vi "Weather Parse Test.vi"() -> ()   [LabVIEW 2020, in "CDM-Config.lvlib"] (continued)
the average of the highest one-\\nthird of the combined wind-wave and swell height.\\n\\n.TONIGHT...NE winds 40 kt. Blowing snow.\\n.WED...NE winds 35 kt.\\n.WED NIGHT...NE winds 30 kt.\\n.THU...NE winds 20 kt.\\n.THU NIGHT...NE winds 20 kt.\\n.FRI...NE winds 20 kt.\\n.FRI NIGHT...NE winds 20 kt.\\n.SAT...NE winds 30 kt.\\n.SUN...NE winds 40 kt.\",\n                \"instruction\": null,\n                \"response\": \"Avoid\",\n                \"parameters\": {\n                    \"AWIPSidentifier\": [\n                        \"CWFWCZ\"\n                    ],\n                    \"WMOidentifier\": [\n                        \"FZAK52 PAFG 030049\"\n                    ],\n                    \"NWSheadline\": [\n                        \"GALE WARNING IN EFFECT THROUGH WEDNESDAY MORNING\"\n                    ],\n                    \"BLOCKCHANNEL\": [\n                        \"EAS\",\n                        \"NWEM\",\n                        \"CMAS\"\n                    ],\n                    \"VTEC\": [\n                        \"/O.NEW.PAFG.GL.W.2010.251203T0000Z-251204T0200Z/\"\n                    ],\n                    \"eventEndingTime\": [\n                        \"2025-12-03T17:00:00-09:00\"\n                    ]\n                },\n                \"scope\": \"Public\",\n                \"code\": \"IPAWSv1.0\",\n                \"language\": \"en-US\",\n                \"web\": \"http://www.weather.gov\",\n                \"eventCode\": {\n                    \"SAME\": [\n                        \"NWS\"\n                    ],\n                    \"NationalWeatherService\": [\n                        \"GLW\"\n                    ]\n                }\n            }\n        },\n        {\n            \"id\": \"https://api.weather.gov/alerts/urn:oid:2.49.0.1.840.0.52fef07b0c3a98d88109cd1837a99c72cb982c5b.007.1\",\n            \"type\": \"Feature\",\n            \"geometry\": null,\n            \"properties\": {\n                \"@id\": \"https://api.weather.gov/alerts/urn:oid:2.49.0.1.840.0.52fef07b0c3a98d88109cd1837a99c72cb982c5b.007.1\",\n                \"@type\": \"wx:Alert\",\n                \"id\": \"urn:oid:2.49.0.1.840.0.52fef07b0c3a98d88109cd1837a99c72cb982c5b.007.1\",\n                \"areaDesc\": \"Wales to Cape Espenberg out to 15 NM\",\n                \"geocode\": {\n                    \"SAME\": [\n                        \"058807\"\n                    ],\n                    \"UGC\": [\n                        \"PKZ807\"\n                    ]\n                },\n                \"affectedZones\": [\n                    \"https://api.weather.gov/zones/forecast/PKZ807\"\n                ],\n                \"references\": [],\n                \"sent\": \"2025-12-02T15:49:00-09:00\",\n                \"effective\": \"2025-12-02T15:49:00-09:00\",\n                \"onset\": \"2025-12-02T15:00:00-09:00\",\n                \"expires\": \"2025-12-03T06:00:00-09:00\",\n                \"ends\": \"2025-12-03T17:00:00-09:00\",\n                \"status\": \"Actual\",\n                \"messageType\": \"Alert\",\n                \"category\": \"Met\",\n                \"severity\": \"Minor\",\n                \"certainty\": \"Likely\",\n                \"urgency\": \"Expected\",\n                \"event\": \"Brisk Wind Advisory\",\n                \"sender\": \"w-nws.webmaster@noaa.gov\",\n                \"senderName\": \"NWS Fairbanks AK\",\n                \"headline\": \"Brisk Wind Advisory issued December 2 at 3:49PM AKST until December 3 at 5:00PM AKST by NWS Fairbanks AK\",\n                \"description\": \"Northwestern Alaska Coastal Waters out 100 NM\\n\\nWind forecasts reflect the predominant speed and direction\\nexpected. Sea forecasts represent the average of the highest one-\\nthird of the combined wind-wave and swell height.\\n\\n.TONIGHT...N winds 30 kt.\\n.WED...N winds 25 kt.\\n.WED NIGHT...SE winds 10 kt.\\n.THU...SE winds 10 kt.\\n.THU NIGHT...E winds 10 kt.\\n.FRI...NE winds 10 kt.\\n.FRI NIGHT...NE winds 15 kt.\\n.SAT...NE winds 25 kt.\\n.SUN...NE winds 30 kt.\",\n                \"instruction\": null,\n                \"response\": \"Avoid\",\n                \"parameters\": {\n                    \"AWIPSidentifier\": [\n                        \"CWFWCZ\"\n                    ],\n                    \"WMOidentifier\": [\n                        \"FZAK52 PAFG 030049\"\n                    ],\n                    \"NWSheadline\": [\n                        \"BRISK WIND ADVISORY IN EFFECT THROUGH WEDNESDAY MORNING\"\n                    ],\n                    \"BLOCKCHANNEL\": [\n                        \"EAS\",\n                        \"NWEM\",\n                        \"CMAS\"\n                    ],\n                    \"VTEC\": [\n                        \"/O.NEW.PAFG.BW.Y.2013.251203T0000Z-251204T0200Z/\"\n                    ],\n                    \"eventEndingTime\": [\n                        \"2025-12-03T17:00:00-09:00\"\n                    ]\n                },\n                \"scope\": \"Public\",\n                \"code\": \"IPAWSv1.0\",\n                \"language\": \"en-US\",\n                \"web\": \"http://www.weather.gov\",\n                \"eventCode\": {\n                    \"SAME\": [\n                        \"NWS\"\n                    ],\n                    \"NationalWeatherService\": [\n                        \"BWY\"\n                    ]\n                }\n            }\n        },\n        {\n            \"id\": \"https://api.weather.gov/alerts/urn:oid:2.49.0.1.840.0.52fef07b0c3a98d88109cd1837a99c72cb982c5b.014.2\",\n            \"type\": \"Feature\",\n            \"geometry\": null,\n            \"properties\": {\n                \"@id\": \"https://api.weather.gov/alerts/urn:oid:2.49.0.1.840.0.52fef07b0c3a98d88109cd1837a99c72cb982c5b.014.2\",\n                \"@type\": \"wx:Alert\",\n                \"id\": \"urn:oid:2.49.0.1.840.0.52fef07b0c3a98d88109cd1837a99c72cb982c5b.014.2\",\n                \"areaDesc\": \"Southwest of Saint Lawrence Island from 15 to 100 NM\",\n                \"geocode\": {\n                    \"SAME\": [\n                        \"058851\"\n                    ],\n                    \"UGC\": [\n                        \"PKZ851\"\n                    ]\n                },\n                \"affectedZones\": [\n                    \"https://api.weather.gov/zones/forecast/PKZ851\"\n                ],\n                \"references\": [],\n                \"sent\": \"2025-12-02T15:49:00-09:00\",\n                \"effective\": \"2025-12-02T15:49:00-09:00\",\n                \"onset\": \"2025-12-02T15:00:00-09:00\",\n                \"expires\": \"2025-12-03T06:00:00-09:00\",\n                \"ends\": \"2025-12-03T17:00:00-09:00\",\n                \"status\": \"Actual\",\n                \"messageType\": \"Alert\",\n                \"category\": \"Met\",\n                \"severity\": \"Severe\",\n                \"certainty\": \"Likely\",\n                \"urgency\": \"Expected\",\n                \"event\": \"Heavy Freezing Spray Warning\",\n                \"sender\": \"w-nws.webmaster@noaa.gov\",\n                \"senderName\": \"NWS Fairbanks AK\",\n                \"headline\": \"Heavy Freezing Spray Warning issued December 2 at 3:49PM AKST until December 3 at 5:00PM AKST by NWS Fairbanks AK\",\n                \"description\": \"Northwestern Alaska Coastal Waters out 100 NM\\n\\nWind forecasts reflect the predominant speed and direction\\nexpected. Sea forecasts represent the average of the highest one-\\nthird of the combined wind-wave and swell height.\\n\\n.TONIGHT...NE winds 40 kt. Seas 13 ft. Heavy freezing spray.\\n.WED...NE winds 35 kt. Seas 10 ft. Heavy freezing spray.\\n.WED NIGHT...N winds 25 kt. Seas 6 ft. Heavy freezing spray.\\n.THU...NE winds 20 kt. Seas 4 ft. Freezing spray.\\n.THU NIGHT...NE winds 20 kt. Seas 4 ft. Heavy freezing spray.\\n.FRI...NE winds 20 kt. Seas 9 ft. Heavy freezing spray.\\n.FRI NIGHT...NE winds 20 kt. Seas 9 ft. Freezing spray.\\n.SAT...NE winds 25 kt. Seas 12 ft.\\n.SUN...NE winds 35 kt. Seas 14 ft.\",\n                \"instruction\": null,\n                \"response\": \"Avoid\",\n                \"parameters\": {\n                    \"AWIPSidentifier\": [\n                        \"CWFWCZ\"\n                    ],\n                    \"WMOidentifier\": [\n                        \"FZAK52 PAFG 030049\"\n                    ],\n                    \"NWSheadline\": [\n                        \"GALE WARNING IN EFFECT THROUGH WEDNESDAY MORNING... ...HEAVY FREEZING SPRAY WARNING IN EFFECT THROUGH WEDNESDAY AFTERNOON\"\n                    ],\n                    \"BLOCKCHANNEL\": [\n                        \"EAS\",\n                        \"NWEM\",\n                        \"CMAS\"\n                    ],\n                    \"VTEC\": [\n                        \"/O.NEW.PAFG.UP.W.2021.251203T0000Z-251204T0200Z/\"\n                    ],\n                    \"eventEndingTime\": [\n                        \"2025-12-03T17:00:00-09:00\"\n                    ]\n                },\n                \"scope\": \"Public\",\n                \"code\": \"IPAWSv1.0\",\n                \"language\": \"en-US\",\n                \"web\": \"http://www.weather.gov\",\n                \"eventCode\": {\n                    \"SAME\": [\n                        \"NWS\"\n                    ],\n                    \"NationalWeatherService\": [\n                        \"UPW\"\n                    ]\n                }\n            }\n        },\n        {\n            \"id\": \"https://api.weather.gov/alerts/urn:oid:2.49.0.1.840.0.52fef07b0c3a98d88109cd1837a99c72cb982c5b.011.1\",\n            \"type\": \"Feature\",\n            \"geometry\": null,\n            \"properties\": {\n                \"@id\": \"https://api.weather.gov/alerts/urn:oid:2.49.0.1.840.0.52fef07b0c3a98d88109cd1837a99c72cb982c5b.011.1\",\n                \"@type\": \"wx:Alert\",\n                \"id\": \"urn:oid:2.49.0.1.840.0.52fef07b0c3a98d88109cd1837a99c72cb982c5b.011.1\",\n                \"areaDesc\": \"South Side of Saint Lawrence Island out to 15 NM\",\n                \"geocode\": {\n                    \"SAME\": [\n                        \"058816\"\n                    ],\n                    \"UGC\": [\n                        \"PKZ816\"\n                    ]\n                },\n                \"affectedZones\": [\n                    \"https://api.weather.gov/zones/forecast/PKZ816\"\n                ],\n                \"references\": [],\n                \"sent\": \"2025-12-02T15:49:00-09:00\",\n                \"effective\": \"2025-12-02T15:49:00-09:00\",\n                \"onset\": \"2025-12-02T15:00:00-09:00\",\n                \"expires\": \"2025-12-03T06:00:00-09:00\",\n                \"ends\": \"2025-12-03T17:00:00-09:00\",\n                \"status\": \"Actual\",\n                \"messageType\": \"Alert\",\n                \"category\": \"Met\",\n                \"severity\": \"Moderate\",\n                \"certainty\": \"Likely\",\n                \"urgency\": \"Expected\",\n                \"event\": \"Gale Warning\",\n                \"sender\": \"w-nws.webmaster@noaa.gov\",\n                \"senderName\": \"NWS Fairbanks AK\",\n                \"headline\": \"Gale Warning issued December 2 at 3:49PM AKST until December 3 at 5:00PM AKST by NWS Fairbanks AK\",\n                \"description\": \"Northwestern Alaska Coastal Waters out 100 NM\\n\\nWind forecasts reflect the predominant speed and direction\\nexpected. Sea forecasts represent the average of the highest one-\\nthird of the combined wind-wave and swell height.\\n\\n.TONIGHT...N winds 40 kt. Seas 10 ft. Heavy freezing spray.\\n.WED...N winds 35 kt. Seas 8 ft. Heavy freezing spray.\\n.WED NIGHT...N winds 25 kt. Seas 5 ft. Heavy freezing spray.\\n.THU...NE winds 15 kt. Seas 3 ft. Freezing spray.\\n.THU NIGHT...NE winds 15 kt. Seas 3 ft. Freezing spray.\\n.FRI...NE winds 15 kt. Seas 6 ft. Heavy freezing spray.\\n.FRI NIGHT...NE winds 20 kt. Seas 8 ft. Freezing spray.\\n.SAT...NE winds 25 kt. Seas 10 ft.\\n.SUN...NE winds 35 kt. Seas 10 ft.\",\n                \"instruction\": null,\n                \"response\": \"Avoid\",\n                \"parameters\": {\n                    \"AWIPSidentifier\": [\n                        \"CWFWCZ\"\n                    ],\n                    \"WMOidentifier\": [\n                        \"FZAK52 PAFG 030049\"\n                    ],\n                    \"NWSheadline\": [\n                        \"GALE WARNING IN EFFECT THROUGH WEDNESDAY MORNING... ...HEAVY FREEZING SPRAY WARNING IN EFFECT THROUGH WEDNESDAY AFTERNOON\"\n                    ],\n                    \"BLOCKCHANNEL\": [\n                        \"EAS\",\n                        \"NWEM\",\n                        \"CMAS\"\n                    ],\n                    \"VTEC\": [\n                        \"/O.NEW.PAFG.GL.W.2014.251203T0000Z-251204T0200Z/\"\n                    ],\n                    \"eventEndingTime\": [\n                        \"2025-12-03T17:00:00-09:00\"\n                    ]\n                },\n                \"scope\": \"Public\",\n                \"code\": \"IPAWSv1.0\",\n                \"language\": \"en-US\",\n                \"web\": \"http://www.weather.gov\",\n                \"eventCode\": {\n                    \"SAME\": [\n                        \"NWS\"\n                    ],\n                    \"NationalWeatherService\": [\n                        \"GLW\"\n                    ]\n                }\n            }\n        },\n        {\n            \"id\": \"https://api.weather.gov/alerts/urn:oid:2.49.0.1.840.0.52fef07b0c3a98d88109cd1837a99c72cb982c5b.006.2\",\n            \"type\": \"Feature\",\n            \"geometry\": null,\n            \"properties\": {\n                \"@id\": \"https://api.weather.gov/alerts/urn:oid:2.49.0.1.840.0.52fef07b0c3a98d88109cd1837a99c72cb982c5b.006.2\",\n                \"@type\": \"wx:Alert\",\n                \"id\": \"urn:oid:2.49.0.1.840.0.52fef07b0c3a98d88109cd1837a99c72cb982c5b.006.2\",\n                \"areaDesc\": \"Sledge Island to Wales out to 15 NM\",\n                \"geocode\": {\n                    \"SAME\": [\n                        \"058806\"\n                    ],\n                    \"UGC\": [\n                        \"PKZ806\"\n                    ]\n                },\n                \"affectedZones\": [\n                    \"https://api.weather.gov/zones/forecast/PKZ806\"\n                ],\n                \"references\": [],\n                \"sent\": \"2025-12-02T15:49:00-09:00\",\n                \"effective\": \"2025-12-02T15:49:00-09:00\",\n                \"onset\": \"2025-12-02T15:00:00-09:00\",\n                \"expires\": \"2025-12-03T06:00:00-09:00\",\n                \"ends\": \"2025-12-03T17:00:00-09:00\",\n                \"status\": \"Actual\",\n                \"messageType\": \"Alert\",\n                \"category\": \"Met\",\n                \"severity\": \"Severe\",\n                \"certainty\": \"Likely\",\n                \"urgency\": \"Expected\",\n                \"event\": \"Heavy Freezing Spray Warning\",\n                \"sender\": \"w-nws.webmaster@noaa.gov\",\n                \"senderName\": \"NWS Fairbanks AK\",\n                \"headline\": \"Heavy Freezing Spray Warning issued December 2 at 3:49PM AKST until December 3 at 5:00PM AKST by NWS Fairbanks AK\",\n                \"description\": \"Northwestern Alaska Coastal Waters out 100 NM\\n\\nWind forecasts reflect the predominant speed and direction\\nexpected. Sea forecasts represent the average of the highest one-\\nthird of the combined wind-wave and swell height.\\n\\n.TONIGHT...N winds 35 kt. Seas 7 ft. Heavy freezing spray.\\n.WED...N winds 35 kt. Seas 6 ft. Heavy freezing spray.\\n.WED NIGHT...NE winds 20 kt. Seas 3 ft. Heavy freezing spray.\\n.THU...NE winds 10 kt. Seas 1 foot.\\n.THU NIGHT...NE winds 10 kt. Seas 2 ft.\\n.FRI...NE winds 15 kt. Seas 3 ft. Heavy freezing spray.\\n.FRI NIGHT...NE winds 20 kt. Seas 5 ft. Heavy freezing spray.\\n.SAT...NE winds 25 kt. Seas 5 ft.\\n.SUN...NE winds 30 kt. Seas 6 ft.\",\n                \"instruction\": null,\n                \"response\": \"Avoid\",\n                \"parameters\": {\n                    \"AWIPSidentifier\": [\n                        \"CWFWCZ\"\n                    ],\n                    \"WMOidentifier\": [\n                        \"FZAK52 PAFG 030049\"\n                    ],\n                    \"NWSheadline\": [\n                        \"GALE WARNING IN EFFECT THROUGH LATE TONIGHT... ...HEAVY FREEZING SPRAY WARNING IN EFFECT THROUGH WEDNESDAY AFTERNOON\"\n                    ],\n                    \"BLOCKCHANNEL\": [\n                        \"EAS\",\n                        \"NWEM\",\n                        \"CMAS\"\n                    ],\n                    \"VTEC\": [\n                        \"/O.NEW.PAFG.UP.W.2012.251203T0000Z-251204T0200Z/\"\n                    ],\n                    \"eventEndingTime\": [\n                        \"2025-12-03T17:00:00-09:00\"\n                    ]\n                },\n                \"scope\": \"Public\",\n                \"code\": \"IPAWSv1.0\",\n                \"language\": \"en-US\",\n                \"web\": \"http://www.weather.gov\",\n                \"eventCode\": {\n                    \"SAME\": [\n                        \"NWS\"\n                    ],\n                    \"NationalWeatherService\": [\n                        \"UPW\"\n                    ]\n                }\n            }\n        },\n        {\n            \"id\": \"https://api.weather.gov/alerts/urn:oid:2.49.0.1.840.0.52fef07b0c3a98d88109cd1837a99c72cb982c5b.012.2\",\n            \"type\": \"Feature\",\n            \"geometry\": null,\n            \"properties\": {\n                \"@id\": \"https://api.weather.gov/alerts/urn:oid:2.49.0.1.840.0.52fef07b0c3a98d88109cd1837a99c72cb982c5b.012.2\",\n                \"@type\": \"wx:Alert\",\n                \"id\": \"urn:oid:2.49.0.1.840.0.52fef07b0c3a98d88109cd1837a99c72cb982c5b.012.2\",\n                \"areaDesc\": \"North Side of Saint Lawrence Island out to 15 NM\",\n                \"geocode\": {\n                    \"SAME\": [\n                        \"058817\"\n                    ],\n                    \"UGC\": [\n                        \"PKZ817\"\n                    ]\n                },\n                \"affectedZones\": [\n                    \"https://api.weather.gov/zones/forecast/PKZ817\"\n                ],\n                \"references\": [],\n                \"sent\": \"2025-12-02T15:49:00-09:00\",\n                \"effective\": \"2025-12-02T15:49:00-09:00\",\n                \"onset\": \"2025-12-02T15:00:00-09:00\",\n                \"expires\": \"2025-12-03T06:00:00-09:00\",\n                \"ends\": \"2025-12-03T17:00:00-09:00\",\n                \"status\": \"Actual\",\n                \"messageType\": \"Alert\",\n                \"category\": \"Met\",\n                \"severity\": \"Severe\",\n                \"certainty\": \"Likely\",\n                \"urgency\": \"Expected\",\n                \"event\": \"Heavy Freezing Spray Warning\",\n                \"sender\": \"w-nws.webmaster@noaa.gov\",\n                \"senderName\": \"NWS Fairbanks AK\",\n                \"headline\": \"Heavy Freezing Spray Warning issued December 2 at 3:49PM AKST until December 3 at 5:00PM AKST by NWS Fairbanks AK\",\n                \"description\": \"Northwestern Alaska Coastal Waters out 100 NM\\n\\nWind forecasts reflect the predominant speed and direction\\nexpected. Sea forecasts represent the average of the highest one-\\nthird of the combined wind-wave and swell height.\\n\\n.TONIGHT...N winds 40 kt. Seas 12 ft. Heavy freezing spray.\\n.WED...N winds 35 kt. Seas 10 ft. Heavy freezing spray.\\n.WED NIGHT...N winds 20 kt. Seas 5 ft. Heavy freezing spray.\\n.THU...NE winds 15 kt. Seas 3 ft.\\n.THU NIGHT...NE winds 10 kt. Seas 2 ft.\\n.FRI...NE winds 20 kt. Seas 6 ft. Freezing spray.\\n.FRI NIGHT...NE winds 20 kt. Seas 9 ft. Heavy freezing spray.\\n.SAT...NE winds 30 kt. Seas 12 ft.\\n.SUN...NE winds 40 kt. Seas 11 ft.\",\n                \"instruction\": null,\n                \"response\": \"Avoid\",\n                \"parameters\": {\n                    \"AWIPSidentifier\": [\n                        \"CWFWCZ\"\n                    ],\n                    \"WMOidentifier\": [\n                        \"FZAK52 PAFG 030049\"\n                    ],\n                    \"NWSheadline\": [\n                        \"GALE WARNING IN EFFECT THROUGH LATE TONIGHT... ...HEAVY FREEZING SPRAY WARNING IN EFFECT THROUGH WEDNESDAY AFTERNOON\"\n                    ],\n                    \"BLOCKCHANNEL\": [\n                        \"EAS\",\n                        \"NWEM\",\n                        \"CMAS\"\n                    ],\n                    \"VTEC\": [\n                        \"/O.NEW.PAFG.UP.W.2017.251203T0000Z-251204T0200Z/\"\n                    ],\n                    \"eventEndingTime\": [\n                        \"2025-12-03T17:00:00-09:00\"\n                    ]\n                },\n                \"scope\": \"Public\",\n                \"code\": \"IPAWSv1.0\",\n                \"language\": \"en-US\",\n                \"web\": \"http://www.weather.gov\",\n                \"eventCode\": {\n                    \"SAME\": [\n                        \"NWS\"\n                    ],\n                    \"NationalWeatherService\": [\n                        \"UPW\"\n                    ]\n                }\n            }\n        },\n        {\n            \"id\": \"https://api.weather.gov/alerts/urn:oid:2.49.0.1.840.0.52fef07b0c3a98d88109cd1837a99c72cb982c5b.019.1\",\n            \"type\": \"Feature\",\n            \"geometry\": null,\n            \"properties\": {\n                \"@id\": \"https://api.weather.gov/alerts/urn:oid:2.49.0.1.840.0.52fef07b0c3a98d88109cd1837a99c72cb982c5b.019.1\",\n                \"@type\": \"wx:Alert\",\n                \"id\": \"urn:oid:2.49.0.1.840.0.52fef07b0c3a98d88109cd1837a99c72cb982c5b.019.1\",\n                \"areaDesc\": \"Wales to Cape Thompson greater than 15 NM\",\n                \"geocode\": {\n                    \"SAME\": [\n                        \"058856\"\n                    ],\n                    \"UGC\": [\n                        \"PKZ856\"\n                    ]\n                },\n                \"affectedZones\": [\n                    \"https://api.weather.gov/zones/forecast/PKZ856\"\n                ],\n                \"references\": [],\n                \"sent\": \"2025-12-02T15:49:00-09:00\",\n                \"effective\": \"2025-12-02T15:49:00-09:00\",\n                \"onset\": \"2025-12-02T15:00:00-09:00\",\n                \"expires\": \"2025-12-03T06:00:00-09:00\",\n                \"ends\": \"2025-12-03T17:00:00-09:00\",\n                \"status\": \"Actual\",\n                \"messageType\": \"Alert\",\n                \"category\": \"Met\",\n                \"severity\": \"Minor\",\n                \"certainty\": \"Likely\",\n                \"urgency\": \"Expected\",\n                \"event\": \"Brisk Wind Advisory\",\n                \"sender\": \"w-nws.webmaster@noaa.gov\",\n                \"senderName\": \"NWS Fairbanks AK\",\n                \"headline\": \"Brisk Wind Advisory issued December 2 at 3:49PM AKST until December 3 at 5:00PM AKST by NWS Fairbanks AK\",\n                \"description\": \"Northwestern Alaska Coastal Waters out 100 NM\\n\\nWind forecasts reflect the predominant speed and direction\\nexpected. Sea forecasts represent the average of the highest one-\\nthird of the combined wind-wave and swell height.\\n\\n.TONIGHT...N winds 25 kt.\\n.WED...N winds 25 kt.\\n.WED NIGHT...S winds 10 kt.\\n.THU...W winds 10 kt.\\n.THU NIGHT...E winds 10 kt.\\n.FRI...NE winds 10 kt.\\n.FRI NIGHT...NE winds 20 kt.\\n.SAT...NE winds 30 kt.\\n.SUN...NE winds 30 kt.\",\n                \"instruction\": null,\n                \"response\": \"Avoid\",\n                \"parameters\": {\n                    \"AWIPSidentifier\": [\n                        \"CWFWCZ\"\n                    ],\n                    \"WMOidentifier\": [\n                        \"FZAK52 PAFG 030049\"\n                    ],\n                    \"NWSheadline\": [\n                        \"BRISK WIND ADVISORY IN EFFECT THROUGH WEDNESDAY MORNING\"\n                    ],\n                    \"BLOCKCHANNEL\": [\n                        \"EAS\",\n                        \"NWEM\",\n                        \"CMAS\"\n                    ],\n                    \"VTEC\": [\n                        \"/O.NEW.PAFG.BW.Y.2026.251203T0000Z-251204T0200Z/\"\n                    ],\n                    \"eventEndingTime\": [\n                        \"2025-12-03T17:00:00-09:00\"\n                    ]\n                },\n                \"scope\": \"Public\",\n                \"code\": \"IPAWSv1.0\",\n                \"language\": \"en-US\",\n                \"web\": \"http://www.weather.gov\",\n                \"eventCode\": {\n                    \"SAME\": [\n                        \"NWS\"\n                    ],\n                    \"NationalWeatherService\": [\n                        \"BWY\"\n                    ]\n                }\n            }\n        },\n        {\n            \"id\": \"https://api.weather.gov/alerts/urn:oid:2.49.0.1.840.0.52fef07b0c3a98d88109cd1837a99c72cb982c5b.013.2\",\n            \"type\": \"Feature\",\n            \"geometry\": null,\n            \"properties\": {\n                \"@id\": \"https://api.weather.gov/alerts/urn:oid:2.49.0.1.840.0.52fef07b0c3a98d88109cd1837a99c72cb982c5b.013.2\",\n                \"@type\": \"wx:Alert\",\n                \"id\": \"urn:oid:2.49.0.1.840.0.52fef07b0c3a98d88109cd1837a99c72cb982c5b.013.2\",\n                \"areaDesc\": \"Etolin Strait to Kwemeluk Pass from 15 to 90 NM\",\n                \"geocode\": {\n                    \"SAME\": [\n                        \"058850\"\n                    ],\n                    \"UGC\": [\n                        \"PKZ850\"\n                    ]\n                },\n                \"affectedZones\": [\n                    \"https://api.weather.gov/zones/forecast/PKZ850\"\n                ],\n                \"references\": [],\n                \"sent\": \"2025-12-02T15:49:00-09:00\",\n                \"effective\": \"2025-12-02T15:49:00-09:00\",\n                \"onset\": \"2025-12-02T15:00:00-09:00\",\n                \"expires\": \"2025-12-03T06:00:00-09:00\",\n                \"ends\": \"2025-12-03T17:00:00-09:00\",\n                \"status\": \"Actual\",\n                \"messageType\": \"Alert\",\n                \"category\": \"Met\",\n                \"severity\": \"Severe\",\n                \"certainty\": \"Likely\",\n                \"urgency\": \"Expected\",\n                \"event\": \"Heavy Freezing Spray Warning\",\n                \"sender\": \"w-nws.webmaster@noaa.gov\",\n                \"senderName\": \"NWS Fairbanks AK\",\n                \"headline\": \"Heavy Freezing Spray Warning issued December 2 at 3:49PM AKST until December 3 at 5:00PM AKST by NWS Fairbanks AK\",\n                \"description\": \"Northwestern Alaska Coastal Waters out 100 NM\\n\\nWind forecasts reflect the predominant speed and direction\\nexpected. Sea forecasts represent the average of the highest one-\\nthird of the combined wind-wave and swell height.\\n\\n.TONIGHT...NE winds 40 kt. Seas 12 ft. Blowing snow. Heavy\\nfreezing spray.\\n.WED...NE winds 35 kt. Seas 10 ft. Heavy freezing spray.\\n.WED NIGHT...NE winds 30 kt. Seas 7 ft. Heavy freezing spray.\\n.THU...NE winds 25 kt. Seas 4 ft. Heavy freezing spray.\\n.THU NIGHT...NE winds 20 kt. Seas 4 ft. Heavy freezing spray.\\n.FRI...NE winds 20 kt. Seas 7 ft. Heavy freezing spray.\\n.FRI NIGHT...NE winds 20 kt. Seas 10 ft. Heavy freezing spray.\\n.SAT...NE winds 25 kt. Seas 12 ft.\\n.SUN...NE winds 35 kt. Seas 12 ft.\",\n                \"instruction\": null,\n                \"response\": \"Avoid\",\n                \"parameters\": {\n                    \"AWIPSidentifier\": [\n                        \"CWFWCZ\"\n                    ],\n                    \"WMOidentifier\": [\n                        \"FZAK52 PAFG 030049\"\n                    ],\n                    \"NWSheadline\": [\n                        \"GALE WARNING IN EFFECT THROUGH WEDNESDAY AFTERNOON... ...HEAVY FREEZING SPRAY WARNING IN EFFECT THROUGH WEDNESDAY AFTERNOON\"\n                    ],\n                    \"BLOCKCHANNEL\": [\n                        \"EAS\",\n                        \"NWEM\",\n                        \"CMAS\"\n                    ],\n                    \"VTEC\": [\n                        \"/O.NEW.PAFG.UP.W.2019.251203T0000Z-251204T0200Z/\"\n                    ],\n                    \"eventEndingTime\": [\n                        \"2025-12-03T17:00:00-09:00\"\n                    ]\n                },\n                \"scope\": \"Public\",\n                \"code\": \"IPAWSv1.0\",\n                \"language\": \"en-US\",\n                \"web\": \"http://www.weather.gov\",\n                \"eventCode\": {\n                    \"SAME\": [\n                        \"NWS\"\n                    ],\n                    \"NationalWeatherService\": [\n                        \"UPW\"\n                    ]\n                }\n            }\n        },\n        {\n            \"id\": \"https://api.weather.gov/alerts/urn:oid:2.49.0.1.840.0.52fef07b0c3a98d88109cd1837a99c72cb982c5b.016.2\",\n            \"type\": \"Feature\",\n            \"geometry\": null,\n            \"properties\": {\n                \"@id\": \"https://api.weather.gov/alerts/urn:oid:2.49.0.1.840.0.52fef07b0c3a98d88109cd1837a99c72cb982c5b.016.2\",\n                \"@type\": \"wx:Alert\",\n                \"id\": \"urn:oid:2.49.0.1.840.0.52fef07b0c3a98d88109cd1837a99c72cb982c5b.016.2\",\n                \"areaDesc\": \"Kwemeluk Pass to Kwikpak Pass from 15 to 90 NM\",\n                \"geocode\": {\n                    \"SAME\": [\n                        \"058853\"\n                    ],\n                    \"UGC\": [\n                        \"PKZ853\"\n                    ]\n                },\n                \"affectedZones\": [\n                    \"https://api.weather.gov/zones/forecast/PKZ853\"\n                ],\n                \"references\": [],\n                \"sent\": \"2025-12-02T15:49:00-09:00\",\n                \"effective\": \"2025-12-02T15:49:00-09:00\",\n                \"onset\": \"2025-12-02T15:00:00-09:00\",\n                \"expires\": \"2025-12-03T06:00:00-09:00\",\n                \"ends\": \"2025-12-03T17:00:00-09:00\",\n                \"status\": \"Actual\",\n                \"messageType\": \"Alert\",\n                \"category\": \"Met\",\n                \"severity\": \"Severe\",\n                \"certainty\": \"Likely\",\n                \"urgency\": \"Expected\",\n                \"event\": \"Heavy Freezing Spray Warning\",\n                \"sender\": \"w-nws.webmaster@noaa.gov\",\n                \"senderName\": \"NWS Fairbanks AK\",\n                \"headline\": \"Heavy Freezing Spray Warning issued December 2 at 3:49PM AKST until December 3 at 5:00PM AKST by NWS Fairbanks AK\",\n                \"description\": \"Northwestern Alaska Coastal Waters out 100 NM\\n\\nWind forecasts reflect the predominant speed and direction\\nexpected. Sea forecasts represent the average of the highest one-\\nthird of the combined wind-wave and swell height.\\n\\n.TONIGHT...N winds 40 kt. Seas 11 ft. Heavy freezing spray.\\n.WED...NE winds 35 kt. Seas 8 ft. Heavy freezing spray.\\n.WED NIGHT...NE winds 25 kt. Seas 5 ft. Heavy freezing spray.\\n.THU...NE winds 15 kt. Seas 3 ft. Heavy freezing spray.\\n.THU NIGHT...NE winds 15 kt. Seas 3 ft. Heavy freezing spray.\\n.FRI...NE winds 15 kt. Seas 5 ft. Heavy freezing spray.\\n.FRI NIGHT...NE winds 20 kt. Seas 8 ft. Heavy freezing spray.\\n.SAT...NE winds 25 kt. Seas 11 ft.\\n.SUN...NE winds 35 kt. Seas 10 ft.\",\n                \"instruction\": null,\n                \"response\": \"Avoid\",\n                \"parameters\": {\n                    \"AWIPSidentifier\": [\n                        \"CWFWCZ\"\n                    ],\n                    \"WMOidentifier\": [\n                        \"FZAK52 PAFG 030049\"\n                    ],\n                    \"NWSheadline\": [\n                        \"GALE WARNING IN EFFECT THROUGH LATE TONIGHT... ...HEAVY FREEZING SPRAY WARNING IN EFFECT THROUGH WEDNESDAY AFTERNOON\"\n                    ],\n                    \"BLOCKCHANNEL\": [\n                        \"EAS\",\n                        \"NWEM\",\n                        \"CMAS\"\n                    ],\n                    \"VTEC\": [\n                        \"/O.NEW.PAFG.UP.W.2023.251203T0000Z-251204T0200Z/\"\n                    ],\n                    \"eventEndingTime\": [\n                        \"2025-12-03T17:00:00-09:00\"\n                    ]\n                },\n                \"scope\": \"Public\",\n                \"code\": \"IPAWSv1.0\",\n                \"language\": \"en-US\",\n                \"web\": \"http://www.weather.gov\",\n                \"eventCode\": {\n                    \"SAME\": [\n                        \"NWS\"\n                    ],\n                    \"NationalWeatherService\": [\n                        \"UPW\"\n                    ]\n                }\n            }\n        },\n        {\n            \"id\": \"https://api.weather.gov/alerts/urn:oid:2.49.0.1.840.0.52fef07b0c3a98d88109cd1837a99c72cb982c5b.017.2\",\n            \"type\": \"Feature\",\n            \"geometry\": null,\n            \"properties\": {\n                \"@id\": \"https://api.weather.gov/alerts/urn:oid:2.49.0.1.840.0.52fef07b0c3a98d88109cd1837a99c72cb982c5b.017.2\",\n                \"@type\": \"wx:Alert\",\n                \"id\": \"urn:oid:2.49.0.1.840.0.52fef07b0c3a98d88109cd1837a99c72cb982c5b.017.2\",\n                \"areaDesc\": \"Sledge Island to Wales greater than 15 NM\",\n                \"geocode\": {\n                    \"SAME\": [\n                        \"058854\"\n                    ],\n                    \"UGC\": [\n                        \"PKZ854\"\n                    ]\n                },\n                \"affectedZones\": [\n                    \"https://api.weather.gov/zones/forecast/PKZ854\"\n                ],\n                \"references\": [],\n                \"sent\": \"2025-12-02T15:49:00-09:00\",\n                \"effective\": \"2025-12-02T15:49:00-09:00\",\n                \"onset\": \"2025-12-02T15:00:00-09:00\",\n                \"expires\": \"2025-12-03T06:00:00-09:00\",\n                \"ends\": \"2025-12-03T17:00:00-09:00\",\n                \"status\": \"Actual\",\n                \"messageType\": \"Alert\",\n                \"category\": \"Met\",\n                \"severity\": \"Severe\",\n                \"certainty\": \"Likely\",\n                \"urgency\": \"Expected\",\n                \"event\": \"Heavy Freezing Spray Warning\",\n                \"sender\": \"w-nws.webmaster@noaa.gov\",\n                \"senderName\": \"NWS Fairbanks AK\",\n                \"headline\": \"Heavy Freezing Spray Warning issued December 2 at 3:49PM AKST until December 3 at 5:00PM AKST by NWS Fairbanks AK\",\n                \"description\": \"Northwestern Alaska Coastal Waters out 100 NM\\n\\nWind forecasts reflect the predominant speed and direction\\nexpected. Sea forecasts represent the average of the highest one-\\nthird of the combined wind-wave and swell height.\\n\\n.TONIGHT...N winds 40 kt. Seas 12 ft. Heavy freezing spray.\\n.WED...N winds 35 kt. Seas 9 ft. Heavy freezing spray.\\n.WED NIGHT...N winds 20 kt. Seas 5 ft. Heavy freezing spray.\\n.THU...N winds 10 kt. Seas 2 ft.\\n.THU NIGHT...NE winds 10 kt. Seas 2 ft.\\n.FRI...NE winds 15 kt. Seas 6 ft. Freezing spray.\\n.FRI NIGHT...NE winds 20 kt. Seas 10 ft. Heavy freezing spray.\\n.SAT...NE winds 30 kt. Seas 12 ft.\\n.SUN...NE winds 35 kt. Seas 10 ft.\",\n                \"instruction\": null,\n                \"response\": \"Avoid\",\n                \"parameters\": {\n                    \"AWIPSidentifier\": [\n                        \"CWFWCZ\"\n                    ],\n                    \"WMOidentifier\": [\n                        \"FZAK52 PAFG 030049\"\n                    ],\n                    \"NWSheadline\": [\n                        \"GALE WARNING IN EFFECT THROUGH LATE TONIGHT... ...HEAVY FREEZING SPRAY WARNING IN EFFECT THROUGH WEDNESDAY AFTERNOON\"\n                    ],\n                    \"BLOCKCHANNEL\": [\n                        \"EAS\",\n                        \"NWEM\",\n                        \"CMAS\"\n                    ],\n                    \"VTEC\": [\n                        \"/O.NEW.PAFG.UP.W.2025.251203T0000Z-251204T0200Z/\"\n                    ],\n                    \"eventEndingTime\": [\n                        \"2025-12-03T17:00:00-09:00\"\n                    ]\n                },\n                \"scope\": \"Public\",\n                \"code\": \"IPAWSv1.0\",\n                \"language\": \"en-US\",\n                \"web\": \"http://www.weather.gov\",\n                \"eventCode\": {\n                    \"SAME\": [\n                        \"NWS\"\n                    ],\n                    \"NationalWeatherService\": [\n                        \"UPW\"\n                    ]\n                }\n            }\n        },\n        {\n            \"id\": \"https://api.weather.gov/alerts/urn:oid:2.49.0.1.840.0.52fef07b0c3a98d88109cd1837a99c72cb982c5b.014.1\",\n            \"type\": \"Feature\",\n            \"geometry\": null,\n            \"properties\": {\n                \"@id\": \"https://api.weather.gov/alerts/urn:oid:2.49.0.1.840.0.52fef07b0c3a98d88109cd1837a99c72cb982c5b.014.1\",\n                \"@type\": \"wx:Alert\",\n                \"id\": \"urn:oid:2.49.0.1.840.0.52fef07b0c3a98d88109cd1837a99c72cb982c5b.014.1\",\n                \"areaDesc\": \"Southwest of Saint Lawrence Island from 15 to 100 NM\",\n                \"geocode\": {\n                    \"SAME\": [\n                        \"058851\"\n                    ],\n                    \"UGC\": [\n                        \"PKZ851\"\n                    ]\n                },\n                \"affectedZones\": [\n                    \"https://api.weather.gov/zones/forecast/PKZ851\"\n                ],\n                \"references\": [],\n                \"sent\": \"2025-12-02T15:49:00-09:00\",\n                \"effective\": \"2025-12-02T15:49:00-09:00\",\n                \"onset\": \"2025-12-02T15:00:00-09:00\",\n                \"expires\": \"2025-12-03T06:00:00-09:00\",\n                \"ends\": \"2025-12-03T17:00:00-09:00\",\n                \"status\": \"Actual\",\n                \"messageType\": \"Alert\",\n                \"category\": \"Met\",\n                \"severity\": \"Moderate\",\n                \"certainty\": \"Likely\",\n                \"urgency\": \"Expected\",\n                \"event\": \"Gale Warning\",\n                \"sender\": \"w-nws.webmaster@noaa.gov\",\n                \"senderName\": \"NWS Fairbanks AK\",\n                \"headline\": \"Gale Warning issued December 2 at 3:49PM AKST until December 3 at 5:00PM AKST by NWS Fairbanks AK\",\n                \"description\": \"Northwestern Alaska Coastal Waters out 100 NM\\n\\nWind forecasts reflect the predominant speed and direction\\nexpected. Sea forecasts represent the average of the highest one-\\nthird of the combined wind-wave and swell height.\\n\\n.TONIGHT...NE winds 40 kt. Seas 13 ft. Heavy freezing spray.\\n.WED...NE winds 35 kt. Seas 10 ft. Heavy freezing spray.\\n.WED NIGHT...N winds 25 kt. Seas 6 ft. Heavy freezing spray.\\n.THU...NE winds 20 kt. Seas 4 ft. Freezing spray.\\n.THU NIGHT...NE winds 20 kt. Seas 4 ft. Heavy freezing spray.\\n.FRI...NE winds 20 kt. Seas 9 ft. Heavy freezing spray.\\n.FRI NIGHT...NE winds 20 kt. Seas 9 ft. Freezing spray.\\n.SAT...NE winds 25 kt. Seas 12 ft.\\n.SUN...NE winds 35 kt. Seas 14 ft.\",\n                \"instruction\": null,\n                \"response\": \"Avoid\",\n                \"parameters\": {\n                    \"AWIPSidentifier\": [\n                        \"CWFWCZ\"\n                    ],\n                    \"WMOidentifier\": [\n                        \"FZAK52 PAFG 030049\"\n                    ],\n                    \"NWSheadline\": [\n                        \"GALE WARNING IN EFFECT THROUGH WEDNESDAY MORNING... ...HEAVY FREEZING SPRAY WARNING IN EFFECT THROUGH WEDNESDAY AFTERNOON\"\n                    ],\n                    \"BLOCKCHANNEL\": [\n                        \"EAS\",\n                        \"NWEM\",\n                        \"CMAS\"\n                    ],\n                    \"VTEC\": [\n                        \"/O.NEW.PAFG.GL.W.2020.251203T0000Z-251204T0200Z/\"\n                    ],\n                    \"eventEndingTime\": [\n                        \"2025-12-03T17:00:00-09:00\"\n                    ]\n                },\n                \"scope\": \"Public\",\n                \"code\": \"IPAWSv1.0\",\n                \"language\": \"en-US\",\n                \"web\": \"http://www.weather.gov\",\n                \"eventCode\": {\n                    \"SAME\": [\n                        \"NWS\"\n                    ],\n                    \"NationalWeatherService\": [\n                        \"GLW\"\n                    ]\n                }\n            }\n        },\n        {\n            \"id\": \"https://api.weather.gov/alerts/urn:oid:2.49.0.1.840.0.8e61c41dab8b41e1fca10497fb00a4c5981d91fc.010.1\",\n            \"type\": \"Feature\",\n            \"geometry\": null,\n            \"properties\": {\n                \"@id\": \"https://api.weather.gov/alerts/urn:oid:2.49.0.1.840.0.8e61c41dab8b41e1fca10497fb00a4c5981d91fc.010.1\",\n                \"@type\": \"wx:Alert\",\n                \"id\": \"urn:oid:2.49.0.1.840.0.8e61c41dab8b41e1fca10497fb00a4c5981d91fc.010.1\",\n                \"areaDesc\": \"Flaxman Island to Demarcation Point from 15 to 75 NM\",\n                \"geocode\": {\n                    \"SAME\": [\n                        \"058861\"\n                    ],\n                    \"UGC\": [\n                        \"PKZ861\"\n                    ]\n                },\n                \"affectedZones\": [\n                    \"https://api.weather.gov/zones/forecast/PKZ861\"\n                ],\n                \"references\": [],\n                \"sent\": \"2025-12-02T15:48:00-09:00\",\n                \"effective\": \"2025-12-02T15:48:00-09:00\",\n                \"onset\": \"2025-12-02T15:00:00-09:00\",\n                \"expires\": \"2025-12-03T06:00:00-09:00\",\n                \"ends\": \"2025-12-03T17:00:00-09:00\",\n                \"status\": \"Actual\",\n                \"messageType\": \"Alert\",\n                \"category\": \"Met\",\n                \"severity\": \"Minor\",\n                \"certainty\": \"Likely\",\n                \"urgency\": \"Expected\",\n                \"event\": \"Brisk Wind Advisory\",\n                \"sender\": \"w-nws.webmaster@noaa.gov\",\n                \"senderName\": \"NWS Fairbanks AK\",\n                \"headline\": \"Brisk Wind Advisory issued December 2 at 3:48PM AKST until December 3 at 5:00PM AKST by NWS Fairbanks AK\",\n                \"description\": \"Arctic Alaska Coastal Waters out 100 NM\\n\\nWind forecasts reflect the predominant speed and direction\\nexpected. Sea forecasts represent the average of the highest one-\\nthird of the combined wind-wave and swell height.\\n\\n.TONIGHT...W winds 25 kt.\\n.WED...W winds 25 kt.\\n.WED NIGHT...W winds 25 kt.\\n.THU...W winds 20 kt.\\n.THU NIGHT...NW winds 10 kt.\\n.FRI...N winds 5 kt.\\n.FRI NIGHT...NE winds 10 kt.\\n.SAT...N winds 10 kt.\\n.SUN...N winds 10 kt.\",\n                \"instruction\": null,\n                \"response\": \"Avoid\",\n                \"parameters\": {\n                    \"AWIPSidentifier\": [\n                        \"CWFNSB\"\n                    ],\n                    \"WMOidentifier\": [\n                        \"FZAK51 PAFG 030048\"\n                    ],\n                    \"NWSheadline\": [\n                        \"BRISK WIND ADVISORY IN EFFECT THROUGH WEDNESDAY AFTERNOON\"\n                    ],\n                    \"BLOCKCHANNEL\": [\n                        \"EAS\",\n                        \"NWEM\",\n                        \"CMAS\"\n                    ],\n                    \"VTEC\": [\n                        \"/O.NEW.PAFG.BW.Y.1842.251203T0000Z-251204T0200Z/\"\n                    ],\n                    \"eventEndingTime\": [\n                        \"2025-12-03T17:00:00-09:00\"\n                    ]\n                },\n                \"scope\": \"Public\",\n                \"code\": \"IPAWSv1.0\",\n                \"language\": \"en-US\",\n                \"web\": \"http://www.weather.gov\",\n                \"eventCode\": {\n                    \"SAME\": [\n                        \"NWS\"\n                    ],\n                    \"NationalWeatherService\": [\n                        \"BWY\"\n                    ]\n                }\n            }\n        },\n        {\n            \"id\": \"https://api.weather.gov/alerts/urn:oid:2.49.0.1.840.0.8e61c41dab8b41e1fca10497fb00a4c5981d91fc.005.1\",\n            \"type\": \"Feature\",\n            \"geometry\": null,\n            \"properties\": {\n                \"@id\": \"https://api.weather.gov/alerts/urn:oid:2.49.0.1.840.0.8e61c41dab8b41e1fca10497fb00a4c5981d91fc.005.1\",\n                \"@type\": \"wx:Alert\",\n                \"id\": \"urn:oid:2.49.0.1.840.0.8e61c41dab8b41e1fca10497fb00a4c5981d91fc.005.1\",\n                \"areaDesc\": \"Flaxman Island to Demarcation Point out to 15 NM\",\n                \"geocode\": {\n                    \"SAME\": [\n                        \"058815\"\n                    ],\n                    \"UGC\": [\n                        \"PKZ815\"\n                    ]\n                },\n                \"affectedZones\": [\n                    \"https://api.weather.gov/zones/forecast/PKZ815\"\n                ],\n                \"references\": [],\n                \"sent\": \"2025-12-02T15:48:00-09:00\",\n                \"effective\": \"2025-12-02T15:48:00-09:00\",\n                \"onset\": \"2025-12-02T15:00:00-09:00\",\n                \"expires\": \"2025-12-03T06:00:00-09:00\",\n                \"ends\": \"2025-12-03T17:00:00-09:00\",\n                \"status\": \"Actual\",\n                \"messageType\": \"Alert\",\n                \"category\": \"Met\",\n                \"severity\": \"Minor\",\n                \"certainty\": \"Likely\",\n                \"urgency\": \"Expected\",\n                \"event\": \"Brisk Wind Advisory\",\n                \"sender\": \"w-nws.webmaster@noaa.gov\",\n                \"senderName\": \"NWS Fairbanks AK\",\n                \"headline\": \"Brisk Wind Advisory issued December 2 at 3:48PM AKST until December 3 at 5:00PM AKST by NWS Fairbanks AK\",\n                \"description\": \"Arctic Alaska Coastal Waters out 100 NM\\n\\nWind forecasts reflect the predominant speed and direction\\nexpected. Sea forecasts represent the average of the highest one-\\nthird of the combined wind-wave and swell height.\\n\\n.TONIGHT...W winds 25 kt.\\n.WED...W winds 25 kt.\\n.WED NIGHT...W winds 25 kt.\\n.THU...W winds 20 kt.\\n.THU NIGHT...NW winds 5 kt.\\n.FRI...NE winds 5 kt.\\n.FRI NIGHT...NE winds 5 kt.\\n.SAT...W winds 10 kt.\\n.SUN...W winds 10 kt.\",\n                \"instruction\": null,\n                \"response\": \"Avoid\",\n                \"parameters\": {\n                    \"AWIPSidentifier\": [\n                        \"CWFNSB\"\n                    ],\n                    \"WMOidentifier\": [\n                        \"FZAK51 PAFG 030048\"\n                    ],\n                    \"NWSheadline\": [\n                        \"BRISK WIND ADVISORY IN EFFECT THROUGH WEDNESDAY AFTERNOON\"\n                    ],\n                    \"BLOCKCHANNEL\": [\n                        \"EAS\",\n                        \"NWEM\",\n                        \"CMAS\"\n                    ],\n                    \"VTEC\": [\n                        \"/O.NEW.PAFG.BW.Y.1841.251203T0000Z-251204T0200Z/\"\n                    ],\n                    \"eventEndingTime\": [\n                        \"2025-12-03T17:00:00-09:00\"\n                    ]\n                },\n                \"scope\": \"Public\",\n                \"code\": \"IPAWSv1.0\",\n                \"language\": \"en-US\",\n                \"web\": \"http://www.weather.gov\",\n                \"eventCode\": {\n                    \"SAME\": [\n                        \"NWS\"\n                    ],\n                    \"NationalWeatherService\": [\n                        \"BWY\"\n                    ]\n                }\n            }\n        },\n        {\n            \"id\": \"https://api.weather.gov/alerts/urn:oid:2.49.0.1.840.0.1f582400c49c338dd966fa4e73bebf0ceb9d5ea9.002.1\",\n            \"type\": \"Feature\",\n            \"geometry\": null,\n            \"properties\": {\n                \"@id\": \"https://api.weather.gov/alerts/urn:oid:2.49.0.1.840.0.1f582400c49c338dd966fa4e73bebf0ceb9d5ea9.002.1\",\n                \"@type\": \"wx:Alert\",\n                \"id\": \"urn:oid:2.49.0.1.840.0.1f582400c49c338dd966fa4e73bebf0ceb9d5ea9.002.1\",\n                \"areaDesc\": \"Cape Suckling to Gravel Point out to 15 NM\",\n                \"geocode\": {\n                    \"SAME\": [\n                        \"058710\"\n                    ],\n                    \"UGC\": [\n                        \"PKZ710\"\n                    ]\n                },\n                \"affectedZones\": [\n                    \"https://api.weather.gov/zones/forecast/PKZ710\"\n                ],\n                \"references\": [],\n                \"sent\": \"2025-12-02T15:47:00-09:00\",\n                \"effective\": \"2025-12-02T15:47:00-09:00\",\n                \"onset\": \"2025-12-03T05:00:00-09:00\",\n                \"expires\": \"2025-12-03T04:45:00-09:00\",\n                \"ends\": \"2025-12-04T05:00:00-09:00\",\n                \"status\": \"Actual\",\n                \"messageType\": \"Alert\",\n                \"category\": \"Met\",\n                \"severity\": \"Minor\",\n                \"certainty\": \"Likely\",\n                \"urgency\": \"Expected\",\n                \"event\": \"Small Craft Advisory\",\n                \"sender\": \"w-nws.webmaster@noaa.gov\",\n                \"senderName\": \"NWS Anchorage AK\",\n                \"headline\": \"Small Craft Advisory issued December 2 at 3:47PM AKST until December 4 at 5:00AM AKST by NWS Anchorage AK\",\n                \"description\": \"Coastal Waters Forecast for the Northern Gulf of Alaska Coast\\nup to 100 nm out including Kodiak Island and Cook Inlet.\\n\\nWind forecasts reflect the predominant speed and direction\\nexpected. Sea forecasts represent an average of the highest\\none-third of the combined wind wave and swell height.\\n\\n.TONIGHT...E wind 30 kt. Seas 10 ft. Rain.\\n.WED...E wind 20 kt. Seas 10 ft. Rain.\\n.WED NIGHT...W wind 15 kt. Seas 9 ft.\\n.THU...Variable wind 10 kt. Seas 8 ft.\\n.THU NIGHT...Variable wind 10 kt. Seas 7 ft.\\n.FRI...E wind 15 kt. Seas 6 ft.\\n.SAT THROUGH SUN...E wind 20 kt. Seas 11 ft.\",\n                \"instruction\": null,\n                \"response\": \"Avoid\",\n                \"parameters\": {\n                    \"AWIPSidentifier\": [\n                        \"CWFAER\"\n                    ],\n                    \"WMOidentifier\": [\n                        \"FZAK51 PAFC 030047\"\n                    ],\n                    \"NWSheadline\": [\n                        \"SMALL CRAFT ADVISORY THROUGH WEDNESDAY NIGHT\"\n                    ],\n                    \"BLOCKCHANNEL\": [\n                        \"EAS\",\n                        \"NWEM\",\n                        \"CMAS\"\n                    ],\n                    \"VTEC\": [\n                        \"/O.NEW.PAFC.SC.Y.7448.251203T1400Z-251204T1400Z/\"\n                    ],\n                    \"eventEndingTime\": [\n                        \"2025-12-04T05:00:00-09:00\"\n                    ]\n                },\n                \"scope\": \"Public\",\n                \"code\": \"IPAWSv1.0\",\n                \"language\": \"en-US\",\n                \"web\": \"http://www.weather.gov\",\n                \"eventCode\": {\n                    \"SAME\": [\n                        \"NWS\"\n                    ],\n                    \"NationalWeatherService\": [\n                        \"SCY\"\n                    ]\n                }\n            }\n        },\n        {\n            \"id\": \"https://api.weather.gov/alerts/urn:oid:2.49.0.1.840.0.1f582400c49c338dd966fa4e73bebf0ceb9d5ea9.005.1\",\n            \"type\": \"Feature\",\n            \"geometry\": null,\n            \"properties\": {\n                \"@id\": \"https://api.weather.gov/alerts/urn:oid:2.49.0.1.840.0.1f582400c49c338dd966fa4e73bebf0ceb9d5ea9.005.1\",\n                \"@type\": \"wx:Alert\",\n                \"id\": \"urn:oid:2.49.0.1.840.0.1f582400c49c338dd966fa4e73bebf0ceb9d5ea9.005.1\",\n                \"areaDesc\": \"Cape Cleare to Gore Point out to 15 NM\",\n                \"geocode\": {\n                    \"SAME\": [\n                        \"058715\"\n                    ],\n                    \"UGC\": [\n                        \"PKZ715\"\n                    ]\n                },\n                \"affectedZones\": [\n                    \"https://api.weather.gov/zones/forecast/PKZ715\"\n                ],\n                \"references\": [],\n                \"sent\": \"2025-12-02T15:47:00-09:00\",\n                \"effective\": \"2025-12-02T15:47:00-09:00\",\n                \"onset\": \"2025-12-03T05:00:00-09:00\",\n                \"expires\": \"2025-12-03T04:45:00-09:00\",\n                \"ends\": \"2025-12-04T05:00:00-09:00\",\n                \"status\": \"Actual\",\n                \"messageType\": \"Alert\",\n                \"category\": \"Met\",\n                \"severity\": \"Minor\",\n                \"certainty\": \"Likely\",\n                \"urgency\": \"Expected\",\n                \"event\": \"Small Craft Advisory\",\n                \"sender\": \"w-nws.webmaster@noaa.gov\",\n                \"senderName\": \"NWS Anchorage AK\",\n                \"headline\": \"Small Craft Advisory issued December 2 at 3:47PM AKST until December 4 at 5:00AM AKST by NWS Anchorage AK\",\n                \"description\": \"Coastal Waters Forecast for the Northern Gulf of Alaska Coast\\nup to 100 nm out including Kodiak Island and Cook Inlet.\\n\\nWind forecasts reflect the predominant speed and direction\\nexpected. Sea forecasts represent an average of the highest\\none-third of the combined wind wave and swell height.\\n\\n.TONIGHT...East wind 20 kt early becoming variable wind 10 kt. Seas\\n8 ft.\\n.WED...Variable wind 10 kt. Seas 8 ft.\\n.WED NIGHT...Variable wind 10 kt. Seas 8 ft.\\n.THU...Variable wind 10 kt. Seas 6 ft.\\n.THU NIGHT...Variable wind 10 kt. Seas 6 ft.\\n.FRI...NE wind 20 kt. Seas 5 ft.\\n.SAT...NE wind 15 kt. Seas 7 ft.\\n.SUN...E wind 15 kt. Seas 11 ft.\",\n                \"instruction\": null,\n                \"response\": \"Avoid\",\n                \"parameters\": {\n                    \"AWIPSidentifier\": [\n                        \"CWFAER\"\n                    ],\n                    \"WMOidentifier\": [\n                        \"FZAK51 PAFC 030047\"\n                    ],\n                    \"NWSheadline\": [\n                        \"SMALL CRAFT ADVISORY THROUGH WEDNESDAY NIGHT\"\n                    ],\n                    \"BLOCKCHANNEL\": [\n                        \"EAS\",\n                        \"NWEM\",\n                        \"CMAS\"\n                    ],\n                    \"VTEC\": [\n                        \"/O.NEW.PAFC.SC.Y.7451.251203T1400Z-251204T1400Z/\"\n                    ],\n                    \"eventEndingTime\": [\n                        \"2025-12-04T05:00:00-09:00\"\n                    ]\n                },\n                \"scope\": \"Public\",\n                \"code\": \"IPAWSv1.0\",\n                \"language\": \"en-US\",\n                \"web\": \"http://www.weather.gov\",\n                \"eventCode\": {\n                    \"SAME\": [\n                        \"NWS\"\n                    ],\n                    \"NationalWeatherService\": [\n                        \"SCY\"\n                    ]\n                }\n            }\n        },\n        {\n            \"id\": \"https://api.weather.gov/alerts/urn:oid:2.49.0.1.840.0.1f582400c49c338dd966fa4e73bebf0ceb9d5ea9.019.1\",\n            \"type\": \"Feature\",\n            \"geometry\": null,\n            \"properties\": {\n                \"@id\": \"https://api.weather.gov/alerts/urn:oid:2.49.0.1.840.0.1f582400c49c338dd966fa4e73bebf0ceb9d5ea9.019.1\",\n                \"@type\": \"wx:Alert\",\n                \"id\": \"urn:oid:2.49.0.1.840.0.1f582400c49c338dd966fa4e73bebf0ceb9d5ea9.019.1\",\n                \"areaDesc\": \"Marmot Island To Sitkinak from 15 to 85 NM\",\n                \"geocode\": {\n                    \"SAME\": [\n                        \"058734\"\n                    ],\n                    \"UGC\": [\n                        \"PKZ734\"\n                    ]\n                },\n                \"affectedZones\": [\n                    \"https://api.weather.gov/zones/forecast/PKZ734\"\n                ],\n                \"references\": [],\n                \"sent\": \"2025-12-02T15:47:00-09:00\",\n                \"effective\": \"2025-12-02T15:47:00-09:00\",\n                \"onset\": \"2025-12-03T05:00:00-09:00\",\n                \"expires\": \"2025-12-03T04:45:00-09:00\",\n                \"ends\": \"2025-12-04T05:00:00-09:00\",\n                \"status\": \"Actual\",\n                \"messageType\": \"Alert\",\n                \"category\": \"Met\",\n                \"severity\": \"Minor\",\n                \"certainty\": \"Likely\",\n                \"urgency\": \"Expected\",\n                \"event\": \"Small Craft Advisory\",\n                \"sender\": \"w-nws.webmaster@noaa.gov\",\n                \"senderName\": \"NWS Anchorage AK\",\n                \"headline\": \"Small Craft Advisory issued December 2 at 3:47PM AKST until December 4 at 5:00AM AKST by NWS Anchorage AK\",\n                \"description\": \"Coastal Waters Forecast for the Northern Gulf of Alaska Coast\\nup to 100 nm out including Kodiak Island and Cook Inlet.\\n\\nWind forecasts reflect the predominant speed and direction\\nexpected. Sea forecasts represent an average of the highest\\none-third of the combined wind wave and swell height.\\n\\n.TONIGHT...SE wind 20 kt. Seas 15 ft. Rain.\\n.WED...S wind 20 kt. Seas 13 ft.\\n.WED NIGHT...SW wind 15 kt. Seas 11 ft.\\n.THU...SE wind 20 kt. Seas 10 ft.\\n.THU NIGHT...E wind 15 kt. Seas 9 ft.\\n.FRI...W wind 20 kt. Seas 9 ft.\\n.SAT THROUGH SUN...W wind 25 kt. Seas 9 ft.\",\n                \"instruction\": null,\n                \"response\": \"Avoid\",\n                \"parameters\": {\n                    \"AWIPSidentifier\": [\n                        \"CWFAER\"\n                    ],\n                    \"WMOidentifier\": [\n                        \"FZAK51 PAFC 030047\"\n                    ],\n                    \"NWSheadline\": [\n                       
